vi "Convert 16xIQData to 16IQpair.vi"(9 "input valid":bool, 10 "16xIQdata in":T2=[{"I"=0.0, "Q"=0.0, "overflow"=FALSE}, {"I"=0.0, "Q"=0.0, "overflow"=FALSE}, {"I"=0.0, "Q"=0.0, "overflow"=FALSE}, {"I"=0.0, "Q"=0.0, "overflow"=FALSE}, {"I"=0.0, "Q"=0.0, "overflow"=FALSE}, {"I"=0.0, "Q"=0.0, "overflow"=FALSE}, {"I"=0.0, "Q"=0.0, "overflow"=FALSE}, {"I"=0.0, "Q"=0.0, "overflow"=FALSE}, {"I"=0.0, "Q"=0.0, "overflow"=FALSE}, {"I"=0.0, "Q"=0.0, "overflow"=FALSE}, {"I"=0.0, "Q"=0.0, "overflow"=FALSE}, {"I"=0.0, "Q"=0.0, "overflow"=FALSE}, {"I"=0.0, "Q"=0.0, "overflow"=FALSE}, {"I"=0.0, "Q"=0.0, "overflow"=FALSE}, {"I"=0.0, "Q"=0.0, "overflow"=FALSE}, {"I"=0.0, "Q"=0.0, "overflow"=FALSE}]) -> (1 "output valid":bool, 2 "16xIQpair out":T1, 5 "Overflow":bool)   [LabVIEW 2015, in "DDC_7976R_v1.lvlib"]
uses:
  DDC_7976R_v1.lvlib
  16xIQData.ctl
  <instrlib>/_niInstr/DSP/v1/Shared/Public/IQ Data.ctl
  16xIQData_without_overflow.ctl
  IQpair_without_overflow.ctl
  <instrlib>/_niInstr/DSP/v1/Shared/niInstr DSP v1 Shared.lvlib
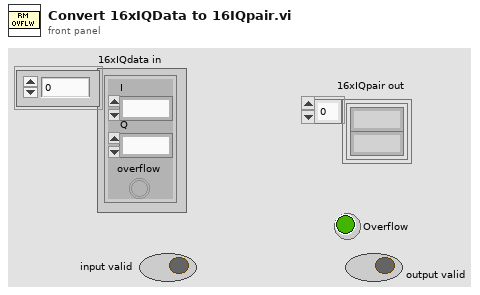
[diagram p1: front panel]
types:
  T1 = typedef "DDC_7976R_v1.lvlib/16xIQData_without_overflow.ctl" = cluster{"I":fxp<+/-,18,1>, "Q":fxp<+/-,18,1>}[]
  T2 = typedef "DDC_7976R_v1.lvlib/16xIQData.ctl" = T3[]
  T3 = typedef "niInstr DSP v1 Shared.lvlib/IQ Data.ctl" = cluster{"I":fxp<+/-,18,1>, "Q":fxp<+/-,18,1>, "overflow":bool}
  T4 = typedef "DDC_7976R_v1.lvlib/IQpair_without_overflow.ctl" = cluster{"I":fxp<+/-,18,1>, "Q":fxp<+/-,18,1>}
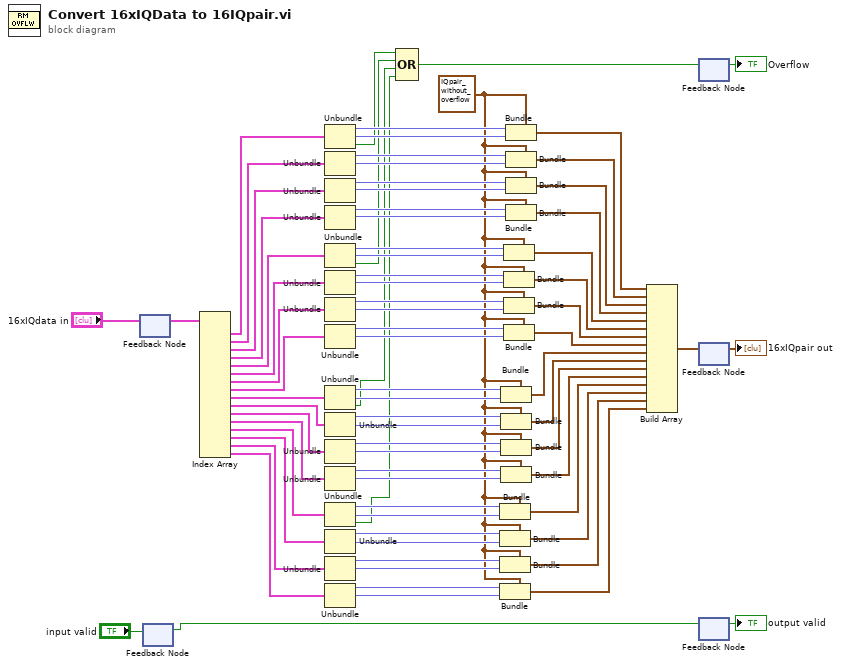
[diagram p0: block diagram]
diagram:
  w30 = T4 {"I"=0.0, "Q"=0.0} ("IQpair wout overflow")
  n1 = feedback-in #1("16xIQdata in") -> ()
  n2 = feedback #1() -> (w8:T2)  [unwired: 1 in]
  n3 = feedback #2() -> (w4:bool)  [unwired: 1 in]
  n4 = feedback-in #2("input valid") -> ()
  n5 = Index Array(array=w8) -> (element #1=w78:T3, element #2=w77:T3, element #3=w76:T3, element #4=w75:T3, element #5=w74:T3, element #6=w73:T3, element #7=w72:T3, element #8=w71:T3, element #9=w70:T3, element #10=w69:T3, element #11=w68:T3, element #12=w67:T3, element #13=w66:T3, element #14=w65:T3, element #15=w64:T3, element #16=w63:T3)  [unwired: 16 in]
  n6 = Unbundle(w78) -> ("I"=w62:fxp<+/-,18,1>, "Q"=w61:fxp<+/-,18,1>, "overflow"=w13:bool)
  n7 = Unbundle(w77) -> ("I"=w60:fxp<+/-,18,1>, "Q"=w59:fxp<+/-,18,1>)  [unwired: 1 out]
  n8 = Unbundle(w76) -> ("I"=w58:fxp<+/-,18,1>, "Q"=w57:fxp<+/-,18,1>)  [unwired: 1 out]
  n9 = Unbundle(w75) -> ("I"=w56:fxp<+/-,18,1>, "Q"=w55:fxp<+/-,18,1>)  [unwired: 1 out]
  n10 = Unbundle(w74) -> ("I"=w54:fxp<+/-,18,1>, "Q"=w53:fxp<+/-,18,1>, "overflow"=w12:bool)
  n11 = Unbundle(w73) -> ("I"=w52:fxp<+/-,18,1>, "Q"=w51:fxp<+/-,18,1>)  [unwired: 1 out]
  n12 = Unbundle(w72) -> ("I"=w50:fxp<+/-,18,1>, "Q"=w49:fxp<+/-,18,1>)  [unwired: 1 out]
  n13 = Unbundle(w71) -> ("I"=w48:fxp<+/-,18,1>, "Q"=w47:fxp<+/-,18,1>)  [unwired: 1 out]
  n14 = Unbundle(w70) -> ("I"=w46:fxp<+/-,18,1>, "Q"=w45:fxp<+/-,18,1>, "overflow"=w11:bool)
  n15 = Unbundle(w69) -> ("I"=w44:fxp<+/-,18,1>, "Q"=w43:fxp<+/-,18,1>)  [unwired: 1 out]
  n16 = Unbundle(w68) -> ("I"=w42:fxp<+/-,18,1>, "Q"=w41:fxp<+/-,18,1>)  [unwired: 1 out]
  n17 = Unbundle(w67) -> ("I"=w40:fxp<+/-,18,1>, "Q"=w39:fxp<+/-,18,1>)  [unwired: 1 out]
  n18 = Unbundle(w66) -> ("I"=w38:fxp<+/-,18,1>, "Q"=w37:fxp<+/-,18,1>, "overflow"=w10:bool)
  n19 = Unbundle(w65) -> ("I"=w36:fxp<+/-,18,1>, "Q"=w35:fxp<+/-,18,1>)  [unwired: 1 out]
  n20 = Unbundle(w64) -> ("I"=w34:fxp<+/-,18,1>, "Q"=w33:fxp<+/-,18,1>)  [unwired: 1 out]
  n21 = Unbundle(w63) -> ("I"=w32:fxp<+/-,18,1>, "Q"=w31:fxp<+/-,18,1>)  [unwired: 1 out]
  n22 = Compound Arithmetic op=OR(w13, w12, w11, w10) -> (w2:bool)
  n23 = Bundle(cluster=w30, "I"=w38, "Q"=w37) -> (w17:T4)
  n24 = Bundle(cluster=w30, "I"=w36, "Q"=w35) -> (w16:T4)
  n25 = Bundle(cluster=w30, "I"=w34, "Q"=w33) -> (w15:T4)
  n26 = Bundle(cluster=w30, "I"=w32, "Q"=w31) -> (w14:T4)
  n27 = Bundle(cluster=w30, "I"=w46, "Q"=w45) -> (w21:T4)
  n28 = Bundle(cluster=w30, "I"=w44, "Q"=w43) -> (w20:T4)
  n29 = Bundle(cluster=w30, "I"=w42, "Q"=w41) -> (w19:T4)
  n30 = Bundle(cluster=w30, "I"=w40, "Q"=w39) -> (w18:T4)
  n31 = Bundle(cluster=w30, "I"=w54, "Q"=w53) -> (w25:T4)
  n32 = Bundle(cluster=w30, "I"=w52, "Q"=w51) -> (w24:T4)
  n33 = Bundle(cluster=w30, "I"=w50, "Q"=w49) -> (w23:T4)
  n34 = Bundle(cluster=w30, "I"=w48, "Q"=w47) -> (w22:T4)
  n35 = Bundle(cluster=w30, "I"=w62, "Q"=w61) -> (w29:T4)
  n36 = Bundle(cluster=w30, "I"=w60, "Q"=w59) -> (w28:T4)
  n37 = Bundle(cluster=w30, "I"=w58, "Q"=w57) -> (w27:T4)
  n38 = Bundle(cluster=w30, "I"=w56, "Q"=w55) -> (w26:T4)
  n39 = Build Array(w29, w28, w27, w26, w25, w24, w23, w22, w21, w20, w19, w18, w17, w16, w15, w14) -> (w6:T4[])
  n40 = feedback #3() -> (→"Overflow":bool)  [unwired: 1 in]
  n41 = feedback-in #3(w2) -> ()
  n42 = feedback #4() -> (→"16xIQpair out":T4[])  [unwired: 1 in]
  n43 = feedback-in #4(w6) -> ()
  n44 = feedback #5() -> (→"output valid":bool)  [unwired: 1 in]
  n45 = feedback-in #5(w4) -> ()
